vi "Get VLIM.vi"(8 "error in (no error)":errorcluster, 11 "SR3XXX HVPS in":refnum<class "SR3XXX HVPS.lvclass">) -> (0 "error out":errorcluster, 2 "V":dbl, 3 "SR3XXX HVPS out":refnum<class "SR3XXX HVPS.lvclass">)   [LabVIEW 2014, in "SR3XXX HVPS.lvclass"]
uses:
  SR3XXX HVPS.lvclass
  reusable/Session APIs/Serial/Typedefs/Session Handle.ctl
  reusable/Session APIs/Serial/Serial Session.lvclass
  Base/Session HVPS.lvclass/Session HVPS.ctl
  Base/Read hSession.vi
  reusable/Session APIs/Serial/Public/Asynchronous Write.vi
  reusable/Session APIs/Serial/Public/Asynchronous Read.vi
  <userlib>/_Session Fwk/Session - Root.lvclass
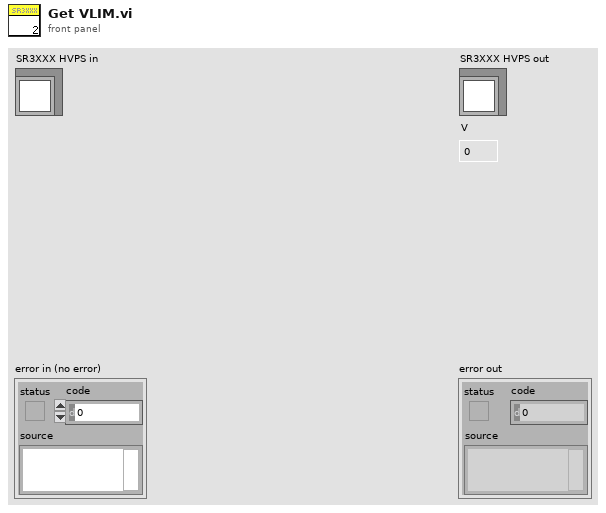
[diagram p1: front panel]
types:
  T1 = typedef "Serial Session.lvclass/Session Handle.ctl" = refnum<data-value>
  T2 = typedef "Session - Root.lvclass/Session Handle.ctl" = refnum<data-value>
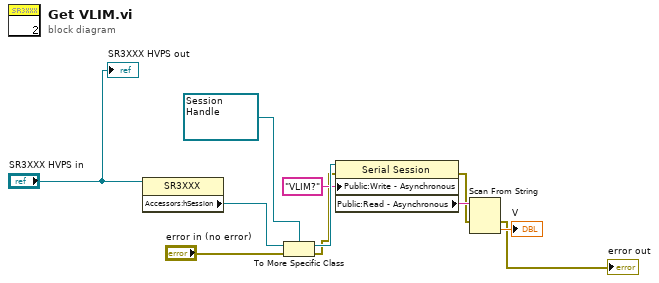
[diagram p0: block diagram]
diagram:
  n1 = property class="SR3XXX"(reference="SR3XXX HVPS in") -> ("Accessors:hSession"=w10:T2)  [unwired: 1 in, 2 out]
  n2 = To More Specific Class(target class=T1 refnum ("Session Handle"), reference=w10, error in="error in (no error)") -> (specific class reference=w8:T1, error out=w3:errorcluster)
  n3 = property class="Serial Session"(reference=w8, error in=w3, "Public:Write - Asynchronous"="VLIM?" ("Cmd")) -> (error out=w2:errorcluster, "Public:Read - Asynchronous"=w6:string)  [unwired: 1 out]
  n4 = Scan From String(input string=w6, error in=w2) -> (error out=→"error out":errorcluster, output 1=→"V":dbl)  [unwired: 3 in, 2 out]
  "SR3XXX HVPS out" <- "SR3XXX HVPS in"
